vi "Error Query.vi"(8 "error in (no error)":errorcluster, 11 "VISA resource name":refnum<visa-resource-name>) -> (0 "error out":errorcluster, 1 "Error Messages":string, 2 "Error Codes":i32[](array[numeric]), 3 "VISA resource name out":refnum<visa-resource-name>)   [LabVIEW 2023, in "Thermotron 8800.lvlib"]
doc: "Queries the instrument for any errors in the instrument's error queue. It will continue to read errors until all errors have been read from the instrument. Any errors will be returned in the <B>error out</B> control.\n\n<B>Note:</B>\nThis VI is called automatically by most driver VIs so it is not usually necessary to call this in an application."
uses:
  Thermotron 8800.lvlib
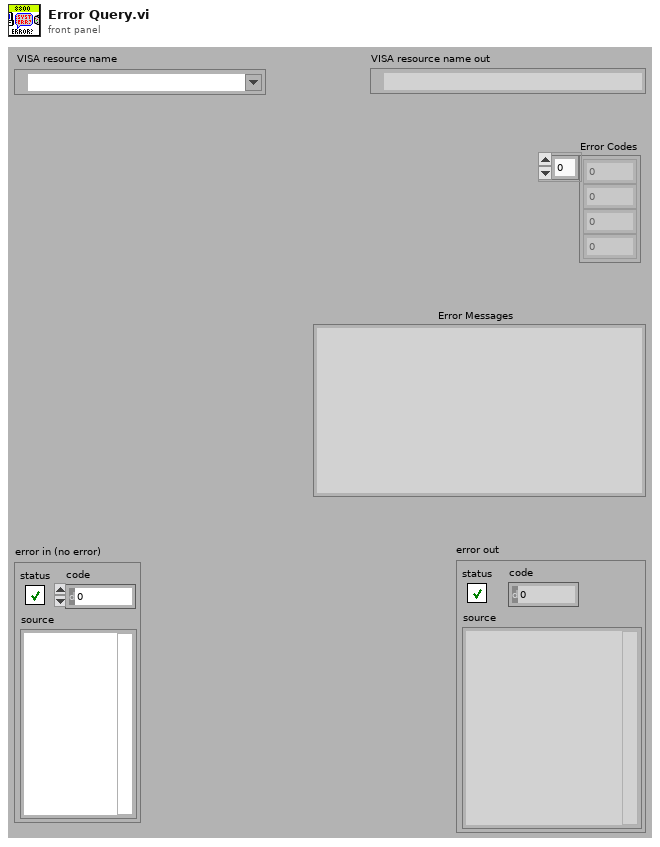
[diagram p1: front panel]
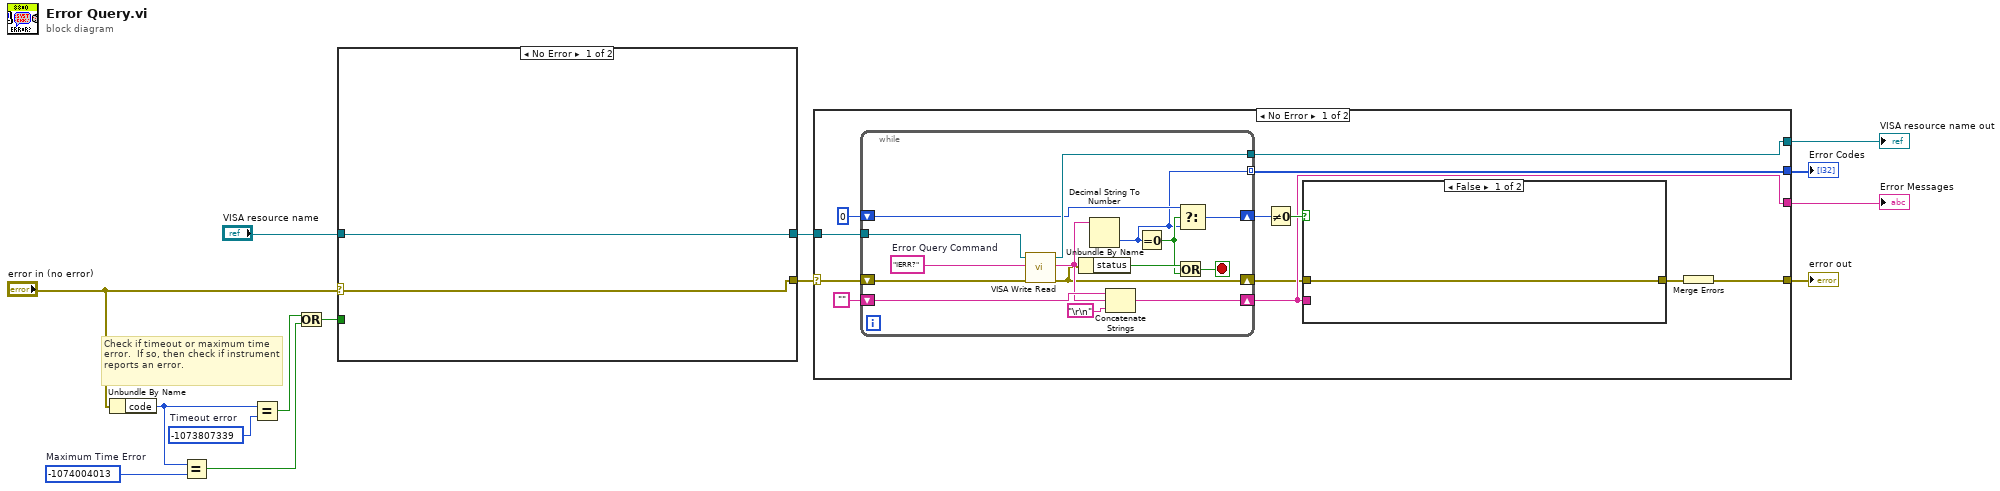
[diagram p0: block diagram]
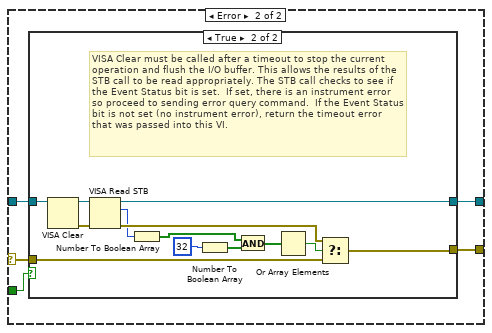
[diagram p2: hidden frame]
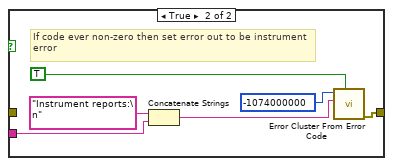
[diagram p4: hidden frame]
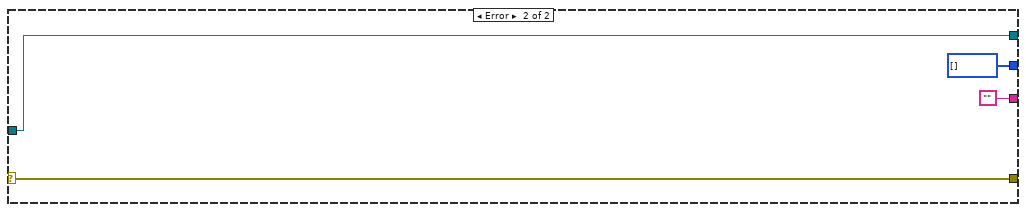
[diagram p5: hidden frame]
diagram:
  w10 = -1074004013  # Maximum Time Error
  w8 = -1073807339  # Timeout error
  # "Check if timeout or maximum time error.  If so, then check if instrument reports an error."
  n1 = Unbundle By Name("error in (no error)") -> ("code"=w9:i32)
  n2 = Equal?(x=w9, y=w10) -> (x = y?=w11:bool)
  n3 = Equal?(x=w9, y=w8) -> (x = y?=w12:bool)
  n4 = Or(x=w12, y=w11) -> (x .or. y?=w13:bool)
  n5 = case shown="No Error" "error in (no error)" {
    selector: "error in (no error)" -> [w15 w19]
    tunnel: "VISA resource name" -> [w16 w21]
    tunnel: [w16 w20] -> w6
    tunnel: [w15 w18] -> w5
    tunnel: w13 -> [_ w17]
    frame No Error {
    }
    frame Error {
      n6 = case shown="True" w17 {
        tunnel: w21 -> [w23 w29]
        tunnel: [w23 w26] -> w20
        tunnel: w19 -> [w22 w32]
        tunnel: [w22 w31] -> w18
        frame False {
          # "Error code not a timeout, so best to pass on to user."
        }
        frame True {
          # "VISA Clear must be called after a timeout to stop the current operation and flush the I/O buffer. This allows the results of the  STB call to be read appropriately. The STB call checks to see if the Event Status bit is set.  If set, there is an instrument error so proceed to sending error query command.  If the Event Status bit is not set (no instrument error), return the timeout error that was passed into this VI."
          n7 = VISA Clear(VISA resource name=w29) -> (VISA resource name out=w28:refnum<visa-resource-name>, error out=w27:errorcluster)  [unwired: 1 in]
          n8 = VISA Read STB(8:w27, 11:w28) -> (0:w25:errorcluster, 2:w24:u16, 3:w26:refnum<visa-resource-name>)
          n9 = Number To Boolean Array(number=w24) -> (Boolean array=w33:bool[])
          n10 = Number To Boolean Array(number=32) -> (Boolean array=w35:bool[])
          n11 = And(x=w33, y=w35) -> (x .and. y?=w34:bool[])
          n12 = Or Array Elements(Boolean array=w34) -> (logical OR=w30:bool)
          n13 = Select(t=w25, s=w30, f=w32) -> (s? t:f=w31:errorcluster)
        }
      }
    }
  }
  n14 = case shown="No Error" w5 {
    selector: w5 -> [w37 w71]
    tunnel: [w48 w74] -> w1
    tunnel: w6 -> [w47 w74]
    tunnel: [w45 w71] -> w2
    tunnel: [w40 ""] -> w3
    tunnel: [w39 i32[] []] -> w4
    frame No Error {
      n15 = while {
        tunnel: [w70] -> w48
        tunnel: w47 -> [w69]
        shift-right: [w66] -> w40
        shift-left: "" -> [w68]
        shift-right: [w64] -> w41
        shift-left: 0 -> [w65]
        shift-right: [w58] -> w38
        shift-left: w37 -> [w63]
        tunnel: [w57] -> w39 mode=indexing
        stop <- w56 stop-if-true
        w60 = "IERR?"  # Error Query Command
        n16 = call "VISA Write Read.vi"("error in (no error)"=w63, "8800 Command"=w60, "VISA Refnum in"=w69) -> ("error out"=w58:errorcluster, "read buffer"=w59:string, "VISA Refnum out"=w70:refnum<visa-resource-name>)  [unwired: 6 in]
        n17 = Unbundle By Name(w58) -> ("status"=w62:bool)
        n18 = Decimal String To Number(string=w59) -> (number=w57:i32)  [unwired: 2 in, 1 out]
        n19 = Concatenate Strings(w68, w59, "\r\n") -> (w66:string)
        n20 = Equal To 0?(x=w57) -> (x = 0?=w61:bool)
        n21 = Or(x=w62, y=w61) -> (x .or. y?=w56:bool)
        n22 = Select(t=w65, s=w61, f=w57) -> (s? t:f=w64:i32)
      }
      n23 = Not Equal To 0?(x=w41) -> (x != 0?=w43:bool)
      n24 = case shown="False" w43 {
        tunnel: w40 -> [_ w54]
        tunnel: [w49 w50] -> w42
        tunnel: w38 -> [w49 _]
        frame False {
        }
        frame True {
          # "If code ever non-zero then set error out to be instrument error"
          n25 = Concatenate Strings("Instrument reports:\n" ("Source"), w54) -> (w51:string)
          n26 = call <vilib>:"Error Cluster From Error Code.vi"("show call chain? (False)"=TRUE, "error message (\"\")"=w51, "error code (0)"=-1074000000 ("Code")) -> ("error out"=w50:errorcluster)  [unwired: 6 in]
        }
      }
      n27 = Merge Errors(w42) -> (w45:errorcluster)
    }
    frame Error {
    }
  }
  "VISA resource name out" <- w1
  "error out" <- w2
  "Error Messages" <- w3
  "Error Codes" <- w4
